vi "SPI Configure.vi"(7 "SPI Channel (0)":u8, 8 "Error In":errorcluster, 10 "SPI Configuration":T1, 11 "LINX Resource":T4) -> (0 "Error Out":errorcluster, 2 "Actual Clock Frequency":u32, 3 "LINX Resource":T4)   [LabVIEW 2011, in "LMH-LINX.lvlib"]
doc: "Configure the specified SPI channel.\n\nClock Frequency: Specify the desired SPI clock frequency. This VI returns the actual achieved clock frequency.\n\nBit Order: Specify the order in which bits are shifted out. \n\nSPI Mode: Chose the SPI mode to determine the clock idle value and sampling edge as follows:\nMode 0 - Clock idle low; data sampled on rising edge.\nMode 1 - Clock idle low; data sampled on faling edge.\nMode 2 - Clock idle high; data sampled on faling edge.\nMode 3 - Clock idle high; data sampled on rising edge."
uses:
  LMH-LINX.lvlib
  Private/Type Defs/LINX Ref.ctl
  Private/Type Defs/Platform.ctl
  Private/Type Defs/Interface.ctl
  Private/Device/Type Defs/LINX Device Config.ctl
  Private/Device/Type Defs/TCP Config.ctl
  Private/Device/Type Defs/Channels.ctl
  Private/Type Defs/Peripherals/SPI/SPI Configuration.ctl
  Private/Type Defs/Peripherals/SPI/SPI Bit Order.ctl
  Private/Type Defs/Peripherals/SPI/SPI Mode.ctl
  Private/Type Defs/Peripheral.ctl
  Private/Type Defs/Channel FGV States.ctl
  Private/Device/Device.lvlib
  <vilib>/myRIO/Common/Instrument Driver Framework/myRIO v1.0/SPI/typedefs/SPI Frame Length.ctl
  <vilib>/myRIO/Common/Instrument Driver Framework/myRIO v1.0/SPI/typedefs/SPI Data Direction.ctl
  <vilib>/myRIO/Common/Instrument Driver Framework/myRIO v1.0/SPI/typedefs/SPI Clock Polarity.ctl
  <vilib>/MakerHub/LINX/Private/Type Defs/Peripherals/SPI/SPI Clock Phase.ctl
  <vilib>/myRIO/Instrument Drivers/Onboard IO/SPI/typedefs/SPI Configuration.ctl
  <vilib>/myRIO/Common/Instrument Driver Framework/myRIO v1.0/SPI/typedefs/SPI Channels Enum.ctl
  <vilib>/myRIO/Common/Instrument Driver Framework/Utilities/typedefs/Generic FPGA Reference.ctl
  <vilib>/myRIO/Common/Instrument Driver Framework/Utilities/typedefs/myRIO v1.0 Reference.ctl
  <vilib>/myRIO/Common/Instrument Driver Framework/Utilities/typedefs/Hardware Version Enum.ctl
  <vilib>/myRIO/Common/Instrument Driver Framework/Utilities/typedefs/myRIO Generic Hardware Reference.ctl
  <vilib>/myRIO/Instrument Drivers/Onboard IO/SPI/typedefs/SPI Reference.ctl
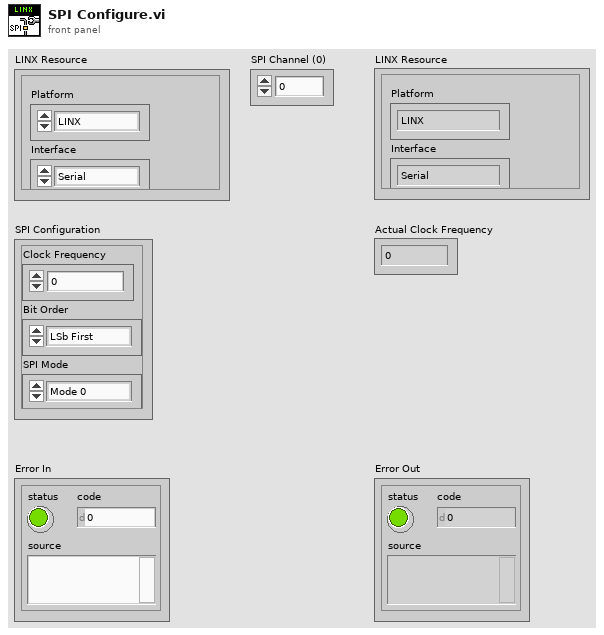
[diagram p1: front panel]
types:
  T1 = typedef "LMH-LINX.lvlib/SPI Configuration.ctl" = cluster{"Clock Frequency":u32, "Bit Order":T2, "SPI Mode":T3}
  T2 = typedef "LMH-LINX.lvlib/SPI Bit Order.ctl" = enum8{"LSb First", "MSb First"}
  T3 = typedef "LMH-LINX.lvlib/SPI Mode.ctl" = enum8{"Mode 0", "Mode 1", "Mode 2", "Mode 3"}
  T4 = typedef "LMH-LINX.lvlib/LINX Ref.ctl" = cluster{"Platform":T5, "Interface":T6, "LINX Device Config":T7}
  T5 = typedef "LMH-LINX.lvlib/Platform.ctl" = enum16{"LINX", "myRIO"}
  T6 = typedef "LMH-LINX.lvlib/Interface.ctl" = enum16{"Serial", "TCP"}
  T7 = typedef "LMH-LINX.lvlib/Device.lvlib/LINX Device Config.ctl" = cluster{"Interface":T6, "COM Port":refnum<visa-resource-name>, "TCP Configuration":T8, "Device Family":u8, "Device ID":u8, "Device Name":string, "TCP Ref":refnum<k5>, "Channels":T9}
  T8 = typedef "LMH-LINX.lvlib/Device.lvlib/TCP Config.ctl" = cluster{"IP Address":string, "Port":u16}
  T9 = typedef "LMH-LINX.lvlib/Channels.ctl" = cluster{"DI":u8[], "DO":u8[], "AI":u8[], "AO":u8[], "PWM":u8[], "QE":u8[], "UART":u8[], "I2C 2":u8[], "SPI":u8[], "CAN":u8[], "Servo":u8[], "AI Ref (V)":dbl, "AO Ref (V)":dbl, "AO Resolution (Bits)":u8}
  T10 = typedef "LMH-LINX.lvlib/Peripheral.ctl" = enum8{"DI", "DO", "AI", "AO", "PWM", "QE", "UART", "I2C", "SPI", "CAN", "Servo"}
  T11 = cluster{"Frequency":dbl, "Clock Phase":u8, "Clock Polarity":u8, "Data Direction":u8, "Frame Length":u8}
  T12 = typedef "LMH-LINX.lvlib/Channel FGV States.ctl" = enum16{"Initialize", "Get", "Set"}
  T13 = typedef "SPI.lvlib/SPI Reference.ctl" = cluster{"myRIO Reference":T14, "SPI Channels Enum":T18, "SPI Configuration":T19}
  T14 = typedef "myRIO Generic Hardware Reference.ctl" = cluster{"myRIO Model":T15, "myRIO Hardware Reference":T16}
  T15 = typedef "Hardware Version Enum.ctl" = enum16{"Unknown", "myRIO-1900", "myRIO-1950"}
  T16 = typedef "myRIO v1.0 Reference.ctl" = cluster{"Generic FPGA Reference":T17, "Allow multiple opens":bool}
  T17 = typedef "Generic FPGA Reference.ctl" = refnum<k20>
  T18 = typedef "SPI Channels Enum.ctl" = enum16{"Not Connected", "A/SPI", "B/SPI"}
  T19 = typedef "SPI.lvlib/SPI Configuration.ctl" = cluster{"Frequency (Hz)":dbl, "Clock Phase":T20, "Clock Polarity":T21, "Data Direction":T22, "Frame Length":T23}
  T20 = typedef "LMH-LINX.lvlib/SPI Clock Phase.ctl" = enum8{"Leading", "Trailing"}
  T21 = typedef "SPI Clock Polarity.ctl" = enum8{"Low", "High"}
  T22 = typedef "SPI Data Direction.ctl" = enum8{"Most Significant Bit First", "Least Significant Bit First"}
  T23 = typedef "SPI Frame Length.ctl" = u8
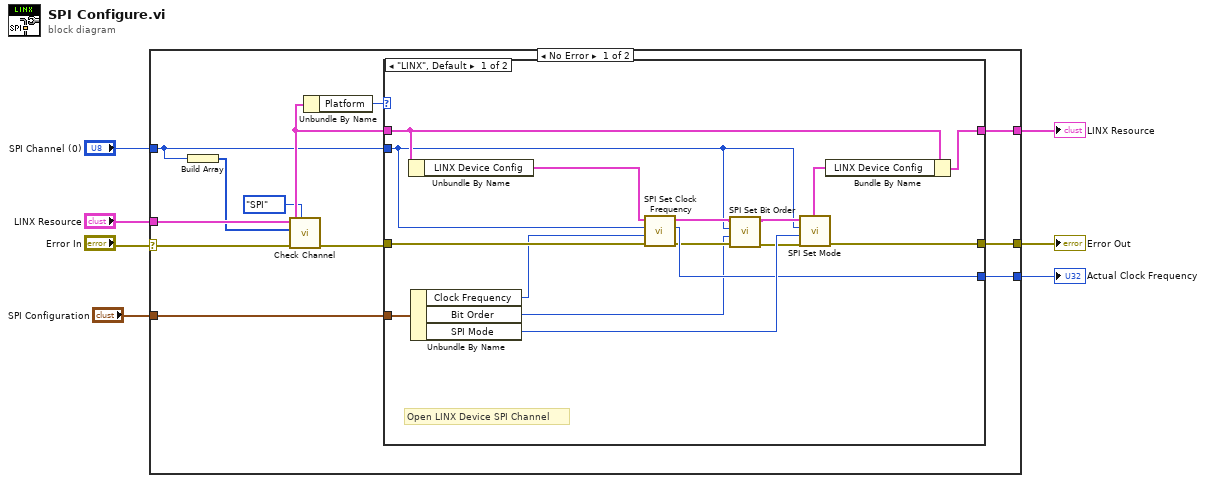
[diagram p0: block diagram]
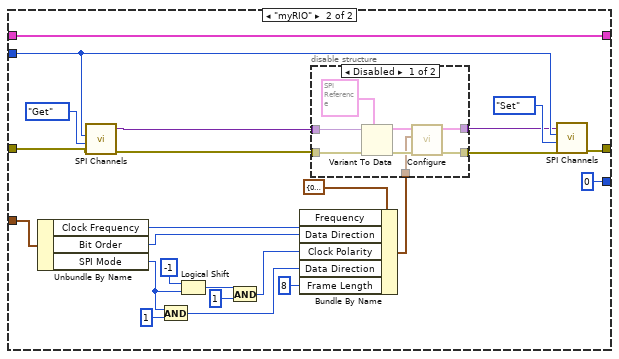
[diagram p2: hidden frame]
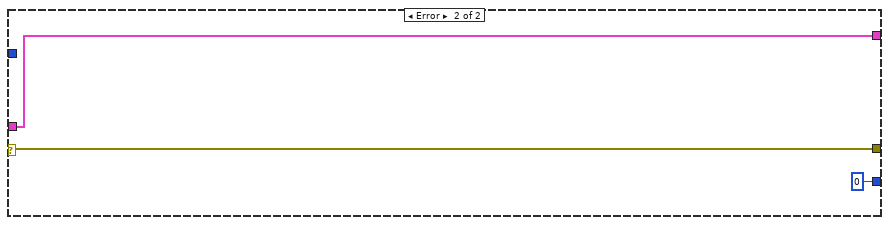
[diagram p4: hidden frame]
diagram:
  n1 = case shown="No Error" "Error In" {
    selector: "Error In" -> [w9 w70]
    tunnel: [w18 w70] -> w7
    tunnel: [w17 w69] -> w6
    tunnel: "LINX Resource" -> [w16 w69]
    tunnel: "SPI Channel (0)" -> [w12 _]
    tunnel: "SPI Configuration" -> [w10 _]
    tunnel: [w8 u32 0 ("Actual Frequency")] -> w1
    frame No Error {
      n2 = Build Array(w12) -> (w13:u8[])
      n3 = call "Check Channel.vi"("Peripheral"=Peripheral."SPI", "Error In"=w9, "Channels"=w13, "LINX Resource"=w16) -> ("Error Out"=w14:errorcluster, "LINX Resource"=w15:T4)  [unwired: 5 in, 1 out]
      n4 = Unbundle By Name(w15) -> ("Platform"=w19:T5)
      n5 = case shown="\"LINX\", Default" w19 {
        tunnel: w14 -> [w29 w56]
        tunnel: w15 -> [w35 w59]
        tunnel: [w31 w58] -> w18
        tunnel: [w34 w59] -> w17
        tunnel: w12 -> [w21 w55]
        tunnel: w10 -> [w33 w53]
        tunnel: [w26 u32 0 ("Actual Frequency")] -> w8
        frame "LINX", Default {
          # "Open LINX Device SPI Channel"
          n6 = Unbundle By Name(w35) -> ("LINX Device Config"=w28:T7)
          n7 = Unbundle By Name(w33) -> ("Clock Frequency"=w27:u32, "Bit Order"=w20:T2, "SPI Mode"=w30:T3)
          n8 = call "SPI Set Clock Frequency.vi"("Error In"=w29, "Target Clock Frequency"=w27, "SPI Channel"=w21, "LINX Device Config"=w28) -> ("Error Out"=w23:errorcluster, "Actual Frequency"=w26:u32, "LINX Device Config"=w25:T7)  [unwired: 5 in]
          n9 = call "SPI Set Bit Order.vi"("Error In"=w23, "SPI Bit Order"=w20, "SPI Channel"=w21, "LINX Device Config"=w25) -> ("Error Out"=w22:errorcluster, "LINX Device Config"=w24:T7)  [unwired: 6 in]
          n10 = call "SPI Set Mode.vi"("Error In"=w22, "SPI Mode"=w30, "SPI Channel"=w21, "LINX Device Config"=w24) -> ("Error Out"=w31:errorcluster, "LINX Device Config"=w32:T7)  [unwired: 6 in]
          n11 = Bundle By Name(cluster=w35, "LINX Device Config"=w32) -> (w34:T4)
        }
        frame "myRIO" {
          n12 = Unbundle By Name(w53) -> ("Clock Frequency"=w49:u32, "Bit Order"=w43:T2, "SPI Mode"=w41:T3)
          n13 = call "SPI Channels.vi"("Error In"=w56, "Channel State"=Channel_FGV_States."Get", "Channel Number"=w55) -> ("Error Out"=w52:errorcluster, "SPI Channel"=w46:variant)  [unwired: 7 in]
          n14 = And(x=w41, y=u8 1 ("Frame Length")) -> (x .and. y?=w42:u8)
          n15 = Logical Shift(y=i8 -1, x=w41) -> (x << y=w38:u32)
          n16 = And(x=w38, y=u8 1 ("Frame Length")) -> (x .and. y?=w37:u32)
          n17 = Bundle By Name(cluster=T11 {"Frequency"=0.0, "Clock Phase"=0, "Clock Polarity"=0, "Data Direction"=0, "Frame Length"=0}, "Frequency"=w49, "Data Direction"=w43, "Clock Polarity"=w37, "Data Direction"=w42, "Frame Length"=u8 8) -> (w45:T11)
          n18 = disable-structure shown="Disabled" {
            disable-tunnel: w52 -> [w64 _]
            disable-tunnel: [w63 _] -> w51
            disable-tunnel: [w62 _] -> w47
            disable-tunnel: w46 -> [w61 _]
            disable-tunnel: w45 -> [w60 _]
            frame Disabled {
              n19 = Variant To Data(error in=w64, type=T13 {"myRIO Reference"={"myRIO Model"=enum."Unknown", "myRIO Hardware Reference"={"Generic FPGA Reference"=refnum, "Allow multiple opens"=FALSE}}, "SPI Channels Enum"=enum."Not Connected", "SPI Configuration"={"Frequency (Hz)"=0.0, "Clock Phase"=enum."Leading", "Clock Polarity"=enum."Low", "Data Direction"=enum."Most Significant Bit First", "Frame Length"=8}} ("SPI Ref In"), Variant=w61) -> (data=w66:T13, error out=w65:errorcluster)
              n20 = call <vilib>:"Configure.vi"("error in (no error)"=w65, "SPI User Configuration"=w60, "SPI Ref In"=w66) -> ("error out"=w63:errorcluster, "SPI Ref Out"=w62:T13)  [unwired: 7 in]
            }
            frame Enabled {
            }
          }
          n21 = call "SPI Channels.vi"("Error In"=w51, "Channel State"=Channel_FGV_States."Set", "Channel Number"=w55, "SPI Channel"=w47) -> ("Error Out"=w58:errorcluster)  [unwired: 6 in, 1 out]
        }
      }
    }
    frame Error {
    }
  }
  "Error Out" <- w7
  "LINX Resource" <- w6
  "Actual Clock Frequency" <- w1
